vi "MOVIE_save_path_folder_definition.vi"(5 "error in":errorcluster, 7 "Sample name":string, 8 "Path to the saving folder":path) -> (0 "error out":errorcluster, 1 "Movie folder":string, 4 "Parameter path":path)   [LabVIEW 2015]
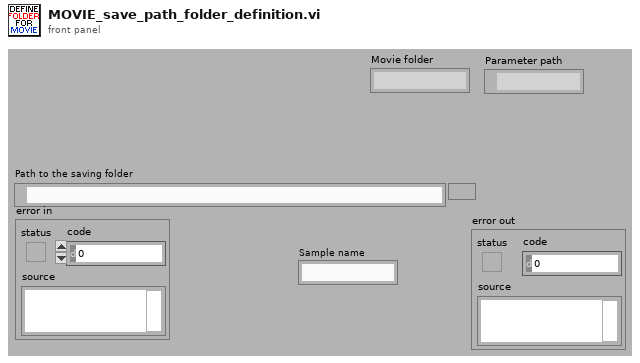
[diagram p1: front panel]
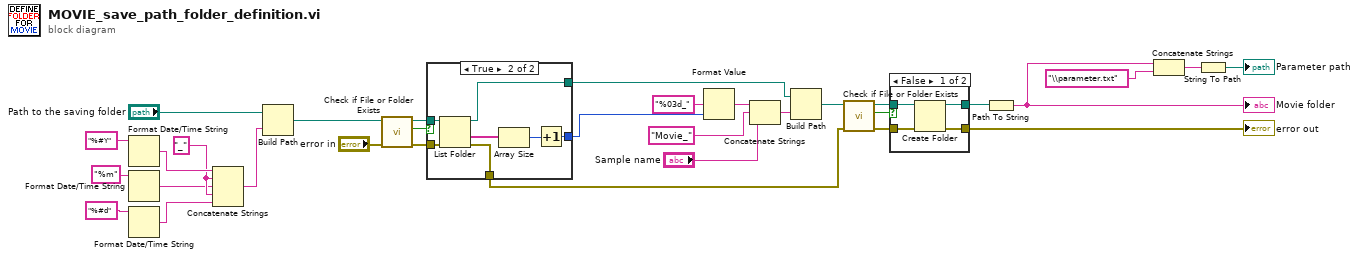
[diagram p0: block diagram]
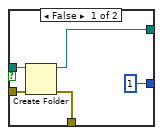
[diagram p3: hidden frame]
diagram:
  w30 = "_" ("string")
  n1 = Format Date/Time String(time format string (%c)="%#Y") -> (date/time string=w31:string)  [unwired: 2 in]
  n2 = Format Date/Time String(time format string (%c)="%m") -> (date/time string=w27:string)  [unwired: 2 in]
  n3 = Format Date/Time String(time format string (%c)="%#d") -> (date/time string=w26:string)  [unwired: 2 in]
  n4 = Concatenate Strings(w31, w30, w27, w30, w26) -> (w24:string)
  n5 = Build Path(base path="Path to the saving folder", name or relative path=w24) -> (appended path=w22:path)
  n6 = call <vilib>:"Check if File or Folder Exists.vi"("error in (no error)"="error in", "path"=w22) -> ("error out"=w7:errorcluster, "file or folder exists?"=w8:bool, "dup path"=w9:path)  [unwired: 7 in]
  n7 = case shown="True" w8 {
    tunnel: w7 -> [w36 w43]
    tunnel: w9 -> [w37 w44]
    tunnel: [w34 w41] -> w12
    tunnel: [w35 w39] -> w10
    tunnel: [1 w42] -> w11
    frame False {
      n8 = Create Folder(path (use dialog)=w37, error in=w36) -> (created path=w34:path, error out=w35:errorcluster)  [unwired: 1 in, 1 out]
    }
    frame True {
      n9 = List Folder(path=w44, error in=w43) -> (path out=w41:path, folder names=w40:string[], error out=w39:errorcluster)  [unwired: 2 in, 1 out]
      n10 = Array Size(array=w40) -> (size(s)=w38:i32)
      n11 = Increment(x=w38) -> (x+1=w42:i32)
    }
  }
  n12 = Format Value(format string="%03d_" ("string (\"\")"), value (0)=w11) -> (output string=w14:string)  [unwired: 1 in]
  n13 = Concatenate Strings(w14, "Movie_" ("string"), "Sample name") -> (w16:string)
  n14 = Build Path(base path=w12, name or relative path=w16) -> (appended path=w17:path)
  n15 = call <vilib>:"Check if File or Folder Exists.vi"("error in (no error)"=w10, "path"=w17) -> ("error out"=w19:errorcluster, "file or folder exists?"=w21:bool, "dup path"=w18:path)  [unwired: 7 in]
  n16 = case shown="False" w21 {
    tunnel: w19 -> [w47 w49]
    tunnel: w18 -> [w48 w50]
    tunnel: [w45 w50] -> w20
    tunnel: [w46 w49] -> w1
    frame False {
      n17 = Create Folder(path (use dialog)=w48, error in=w47) -> (created path=w45:path, error out=w46:errorcluster)  [unwired: 1 in, 1 out]
    }
    frame True {
    }
  }
  "error out" <- w1
  n18 = Path To String(path=w20) -> (string=w5:string)
  "Movie folder" <- w5
  n19 = Concatenate Strings(w5, "\\parameter.txt" ("string")) -> (w2:string)
  n20 = String To Path(string=w2) -> (path=→"Parameter path":path)
